vi "Write Ring Control.vi"(8 "error in":errorcluster, 10 "Value":string[](array[string]), 11 "Ring Control Ref in":refnum<vi>) -> (0 "error out":errorcluster, 3 "Ring Control Ref out":refnum<vi>)   [LabVIEW 2020, in "G-Unicode.lvlib"]
uses:
  G-Unicode.lvlib
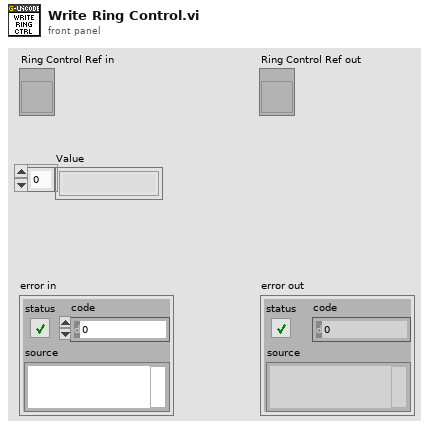
[diagram p1: front panel]
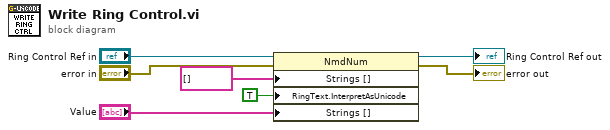
[diagram p0: block diagram]
diagram:
  n1 = property class="NmdNum"(reference="Ring Control Ref in", error in="error in", "Strings []"=string[] [], "RingText.InterpretAsUnicode"=TRUE ("Ring Text.Interpret As Unicode"), "Strings []"="Value") -> (reference out=→"Ring Control Ref out":refnum<vi>, error out=→"error out":errorcluster)
